vi "Destroy.vi"(8 "error in (no error)":errorcluster, 11 "Thread":refnum<class "Thread.lvclass">) -> (0 "error out":errorcluster, 3 "Thread type":refnum<class "Thread.lvclass">)   [LabVIEW 2017, in "DSF Core.lvlib" / "Thread.lvclass"]
uses:
  Thread.lvclass
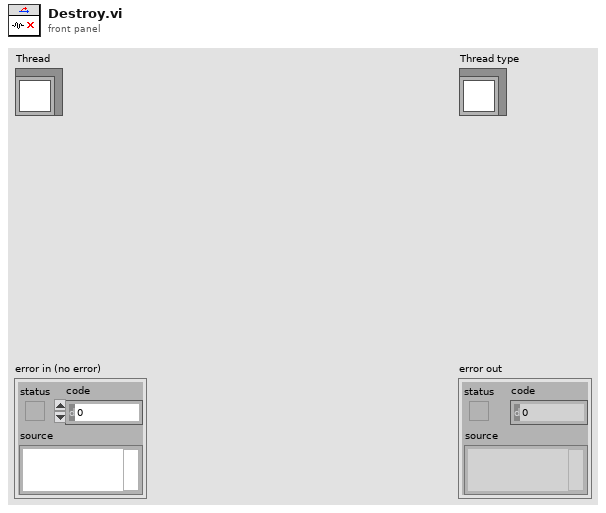
[diagram p1: front panel]
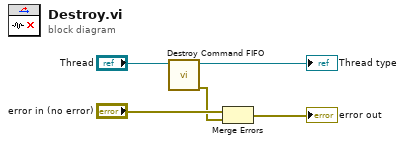
[diagram p0: block diagram]
diagram:
  n1 = call "Destroy Command FIFO.vi"("Thread in"="Thread") -> ("error out"=w2:errorcluster, "Thread out"=→"Thread type":refnum<class "Thread.lvclass">)  [unwired: 9 in]
  n2 = Merge Errors("error in (no error)", w2) -> (→"error out":errorcluster)
